vi "Write Resource.vi"(8 "error in (no error)":errorcluster, 10 "Resource":string, 11 "Digital Delay Generator in":refnum<class "Digital Delay Generator.lvclass">) -> (0 "error out":errorcluster, 3 "Digital Delay Generator out":refnum<class "Digital Delay Generator.lvclass">)   [LabVIEW 2018, in "Digital Delay Generator.lvlib" / "Digital Delay Generator.lvclass"]
uses:
  Digital Delay Generator.lvclass
  Digital Delay Generator.lvclass/Digital Delay Generator.ctl
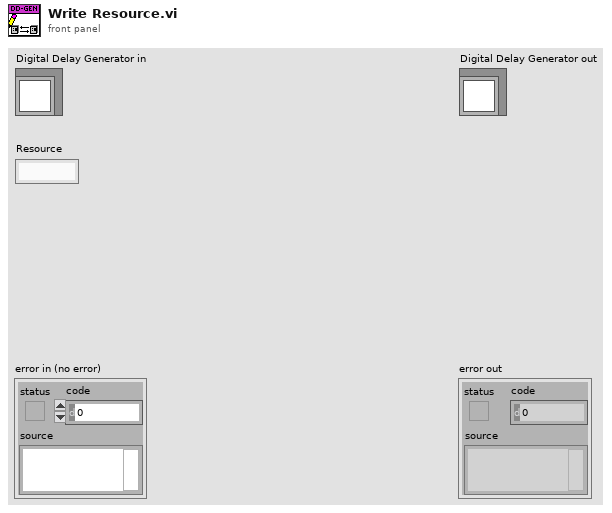
[diagram p1: front panel]
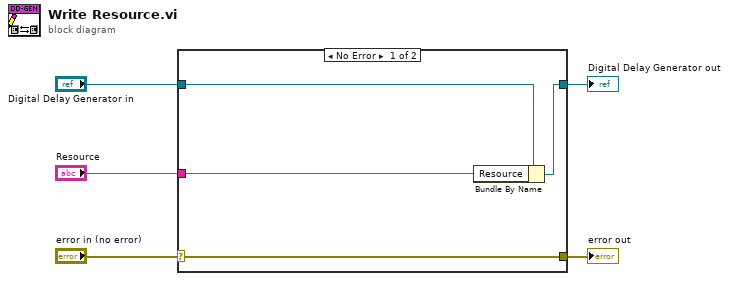
[diagram p0: block diagram]
diagram:
  n1 = case shown="No Error" "error in (no error)" {
    selector: "error in (no error)" -> [w9 w10]
    tunnel: [w9 w10] -> w4
    tunnel: [w7 w11] -> w2
    tunnel: "Digital Delay Generator in" -> [w8 w11]
    tunnel: "Resource" -> [w6 _]
    frame No Error {
      n2 = Bundle By Name(cluster=w8, "Resource"=w6) -> (w7:refnum<class "Digital Delay Generator.lvclass">)
    }
    frame Error {
    }
  }
  "error out" <- w4
  "Digital Delay Generator out" <- w2
